vi "Read Storage Account URI.vi"(8 "error in (no error)":errorcluster, 11 "Azure Session in":refnum<class "Session.lvclass">) -> (0 "error out":errorcluster, 2 "Storage Account URI":string, 3 "Azure Session out":refnum<class "Session.lvclass">)   [LabVIEW 2015, in "NI_Azure_Core.lvlib" / "Session.lvclass"]
uses:
  Session.lvclass
  Session.lvclass/Session.ctl
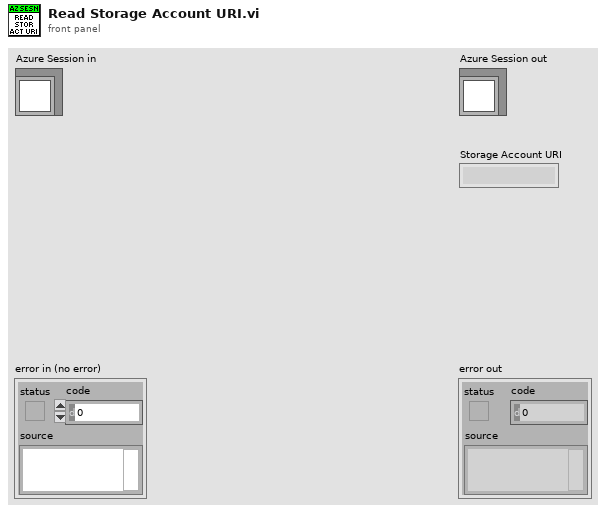
[diagram p1: front panel]
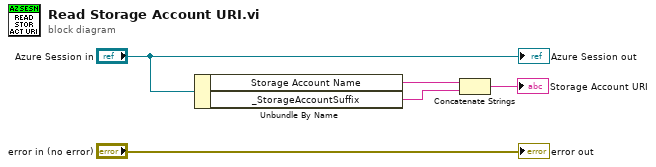
[diagram p0: block diagram]
diagram:
  n1 = Unbundle By Name("Azure Session in") -> ("Storage Account Name"=w3:string, "_StorageAccountSuffix"=w2:string)
  n2 = Concatenate Strings(w3, w2) -> (→"Storage Account URI":string)
  "error out" <- "error in (no error)"
  "Azure Session out" <- "Azure Session in"
